vi "Read Spectrum and Save It_OK.vi"(0 "VISA Session":refnum<visa-resource-name>="GPIB1::9::INSTR", 6 "Pasta Destino DESTA aquisicao":path, 9 "Corrente Atual (mA)":dbl, 11 "Error In":errorcluster, 12 "Iteracao":i32) -> (2 "X":dbl[](array[numeric]) format="%.12f", 3 "Y":dbl[](array[numeric]) format="%.12f", 4 "Copy VISA Session":refnum<visa-resource-name>, 8 "PxI":dbl[](array[numeric]), 10 "XY Graph":T1(graph), 14 "PxLambda":dbl[](array[numeric]), 15 "Error Out":errorcluster)   [LabVIEW 2021]
panel:
  out "Return Data Bytes 2":u16
  out "Wavelike Data (X)":dbl[](array[numeric]) format="%.12f"
  out "Return All Data 2":string
  out "Wavelike Data (Y)":dbl[](array[numeric]) format="%.12f"
  out "Return Data Bytes":u16
  out "Return All Data":string
  # "Antes de utilizar esta VI, deve-se executar a VI de configuração do espectrômetro antes (Config Spectrometer.vi)."
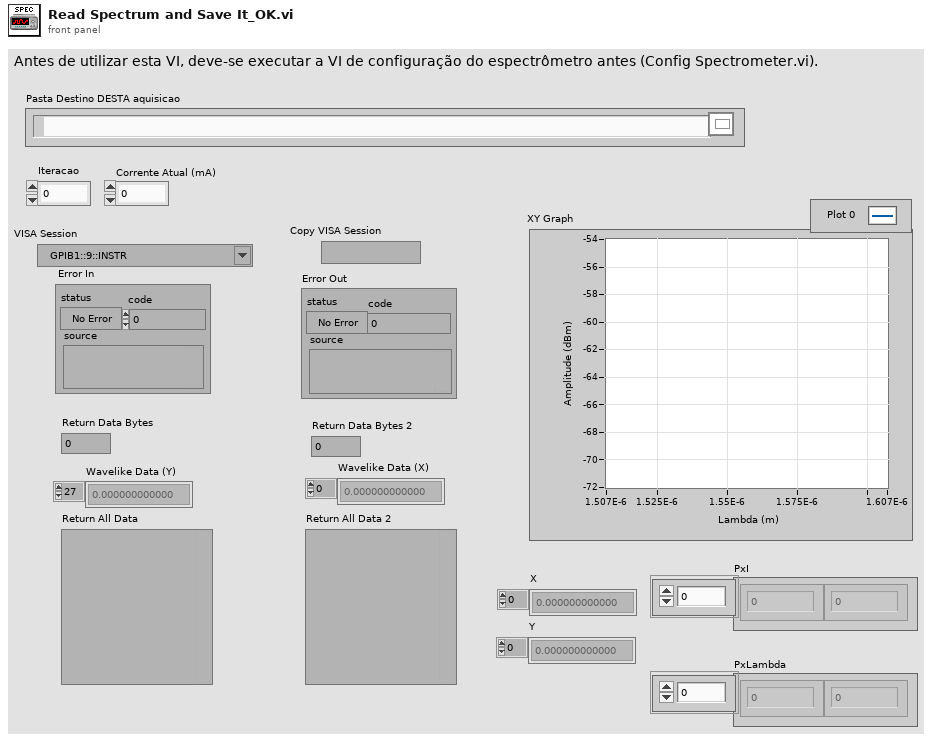
[diagram p1: front panel]
types:
  T1 = cluster{"Wavelike Data":dbl[], "Wavelike Data":dbl[]}
  T2 = enum16{"Y AXIS Data Output", "X AXIS Data Output"}
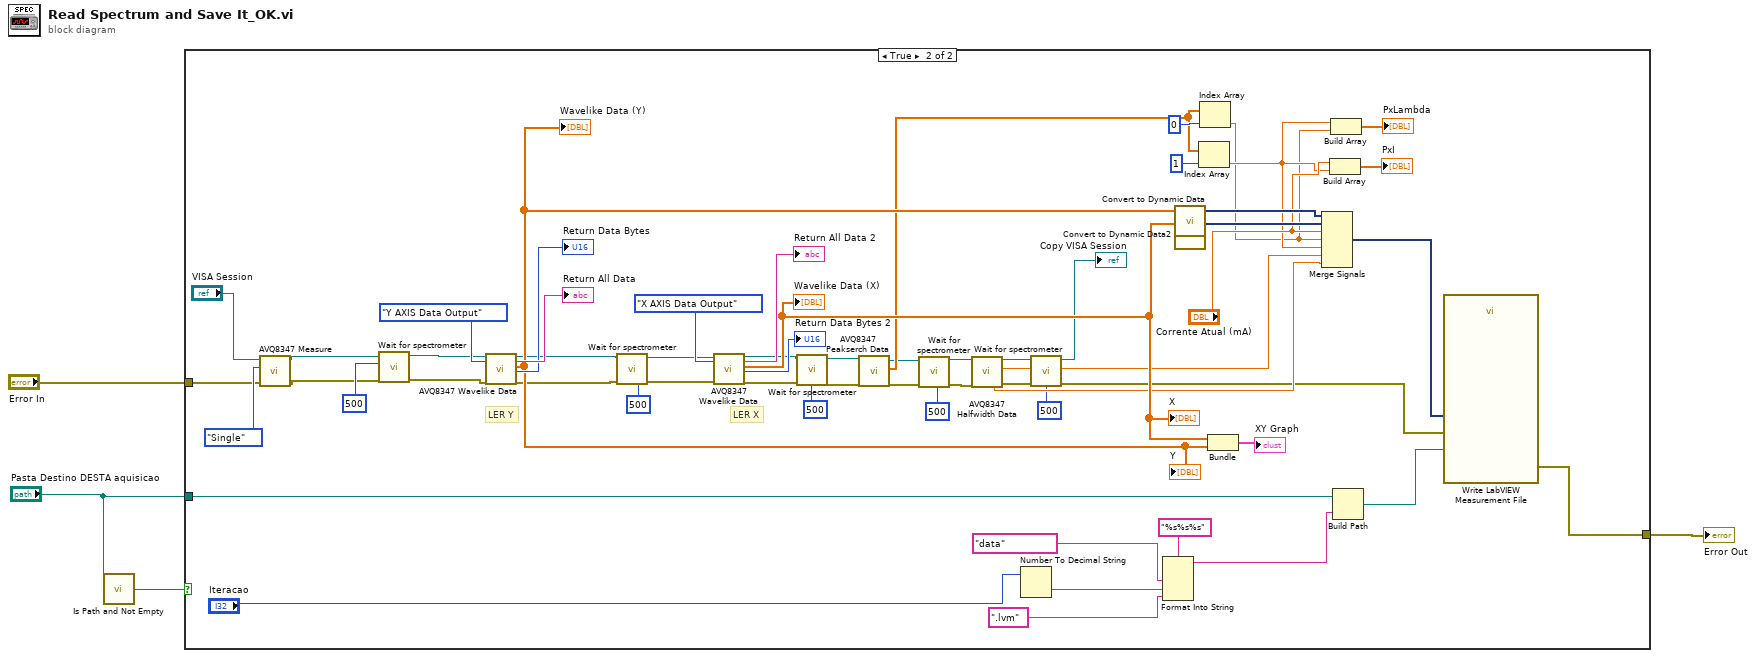
[diagram p0: block diagram]
diagram:
  n1 = call <vilib>:"Is Path and Not Empty.vi"("path"="Pasta Destino DESTA aquisicao") -> ("Is Path and Not Empty?"=w3:bool)  [unwired: 4 in]
  n2 = case shown="True" w3 {
    tunnel: "Pasta Destino DESTA aquisicao" -> [_ w55]
    tunnel: "Error In" -> [w5 w41]
    tunnel: [w5 w40] -> w1
    frame False {
    }
    frame True {
      # "LER X"
      # "LER Y"
      n3 = call "AVQ8347 Measure.vi"("Error In"=w41, "Measure Select"=enum16{"Stop", "Single", "Repeat"}."Single", "VISA Session"="VISA Session") -> ("Error Out"=w24:errorcluster, "Copy VISA Session"=w25:refnum<visa-resource-name>)  [unwired: 6 in, 1 out]
      n4 = call "Wait for spectrometer.vi"("error in (no error)"=w24, "milliseconds to wait"=u32 500, "VISA Refnum in"=w25) -> ("error out"=w46:errorcluster, "VISA Refnum out"=w47:refnum<visa-resource-name>)  [unwired: 6 in, 1 out]
      n5 = call "AVQ8347 Wavelike Data.vi"("VISA Session"=w47, "Axis Select"=T2."Y AXIS Data Output", "Error In"=w46) -> ("Copy VISA Session"=w30:refnum<visa-resource-name>, "Return All Data"=→"Return All Data":string, "Wavelike Data"=w53:dbl[], "Return Data Bytes"=→"Return Data Bytes":u16, "Error Out"=w42:errorcluster)  [unwired: 12 in]
      "Wavelike Data (Y)" <- w53
      "Y" <- w53
      n6 = call "Wait for spectrometer.vi"("error in (no error)"=w42, "milliseconds to wait"=u32 500, "VISA Refnum in"=w30) -> ("error out"=w43:errorcluster, "VISA Refnum out"=w44:refnum<visa-resource-name>)  [unwired: 6 in, 1 out]
      n7 = call "AVQ8347 Wavelike Data.vi"("VISA Session"=w44, "Axis Select"=T2."X AXIS Data Output", "Error In"=w43) -> ("Copy VISA Session"=w29:refnum<visa-resource-name>, "Return All Data"=→"Return All Data 2":string, "Wavelike Data"=w54:dbl[], "Return Data Bytes"=→"Return Data Bytes 2":u16, "Error Out"=w39:errorcluster)  [unwired: 12 in]
      "Wavelike Data (X)" <- w54
      "X" <- w54
      n8 = call "Wait for spectrometer.vi"("error in (no error)"=w39, "milliseconds to wait"=u32 500, "VISA Refnum in"=w29) -> ("error out"=w36:errorcluster, "VISA Refnum out"=w37:refnum<visa-resource-name>)  [unwired: 6 in, 1 out]
      n9 = call "AVQ8347 Peakserch Data.vi"("VISA Session"=w37, "Error In"=w36) -> ("Copy VISA Session"=w16:refnum<visa-resource-name>, "Peakserch Data"=w33:dbl[], "Error Out"=w15:errorcluster)  [unwired: 13 in, 2 out]
      n10 = call "Wait for spectrometer.vi"("error in (no error)"=w15, "milliseconds to wait"=u32 500, "VISA Refnum in"=w16) -> ("error out"=w11:errorcluster, "VISA Refnum out"=w12:refnum<visa-resource-name>)  [unwired: 6 in, 1 out]
      n11 = call "AVQ8347 Halfwidth Data.vi"("VISA Session"=w12, "Error In"=w11) -> ("Fitting Error"=w17:dbl, "Copy VISA Session"=w10:refnum<visa-resource-name>, "HalfWidth"=w18:dbl, "Error Out"=w9:errorcluster)  [unwired: 10 in, 4 out]
      n12 = Number To Decimal String(number="Iteracao") -> (decimal integer string=w28:string)  [unwired: 1 in]
      n13 = call "Wait for spectrometer.vi"("error in (no error)"=w9, "milliseconds to wait"=u32 500, "VISA Refnum in"=w10) -> ("error out"=w7:errorcluster, "VISA Refnum out"=→"Copy VISA Session":refnum<visa-resource-name>)  [unwired: 6 in, 1 out]
      n14 = Format Into String(format string="%s%s%s", "data", w28, ".lvm") -> (resulting string=w49:string)  [unwired: 2 in, 1 out]
      n15 = call "Convert to Dynamic Data"("Array"=w53) -> ("Dynamic Data Type"=w57:dynamicdata)  [unwired: 3 in]
      n16 = call "Convert to Dynamic Data2"("Array"=w54) -> ("Dynamic Data Type"=w56:dynamicdata)  [unwired: 3 in]
      n17 = Index Array(array=w33, index=1) -> (element=w21:dbl)
      n18 = Index Array(array=w33, index=0) -> (element=w20:dbl)
      n19 = Bundle("Wavelike Data"=w54, "Wavelike Data"=w53) -> (→"XY Graph":T1)  [unwired: 1 in]
      n20 = Merge Signals(w57, w56, "Corrente Atual (mA)", w20, w21, w18, w17) -> (w58:dynamicdata)
      n21 = Build Array("Corrente Atual (mA)", w21) -> (→"PxI":dbl[])
      n22 = Build Array(w21, w20) -> (→"PxLambda":dbl[])
      n23 = Build Path(base path=w55, name or relative path=w49) -> (appended path=w38:path)
      n24 = call "Write LabVIEW Measurement File"("Signals"=w58, "error in (no error)"=w7, "Filename"=w38) -> ("error out"=w40:errorcluster)  [unwired: 14 in, 2 out]
    }
  }
  "Error Out" <- w1
